vi "Global Stop Actions.vi"(7 "Command":T2=enum."Read", 8 "error in (no error)":errorcluster, 9 "Stop on Error?":bool, 10 "Stop?":bool, 11 "Stop Ref":T1) -> (0 "error out":errorcluster {"code" min=0 max=0}, 2 "Latched Stop":bool, 3 "Stop Ref out":T1)   [LabVIEW 2013, in "J1939 Addon Engine.lvlib" / "Stop FG.lvlib"]
uses:
  Stop FG.lvlib
  Stop Global Ref.ctl
  Stop Global Commands.ctl
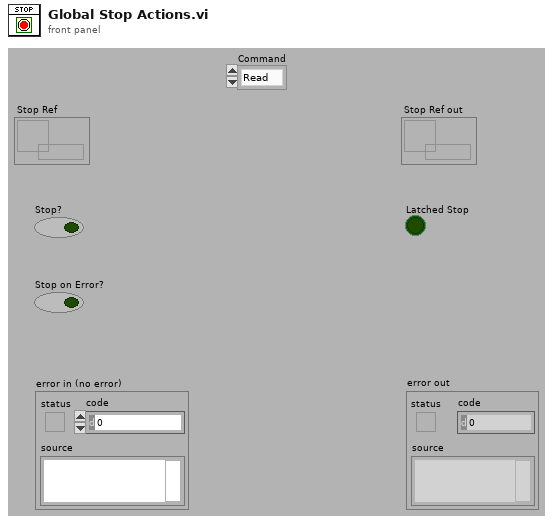
[diagram p1: front panel]
types:
  T1 = typedef "J1939 Addon Engine.lvlib/Stop FG.lvlib/Stop Global Ref.ctl" = refnum<data-value>
  T2 = typedef "J1939 Addon Engine.lvlib/Stop FG.lvlib/Stop Global Commands.ctl" = enum16{"Write", "Read", "Reset"}
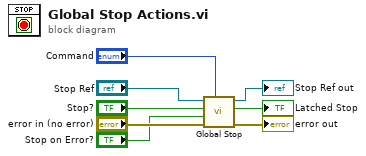
[diagram p0: block diagram]
diagram:
  n1 = call "Global Stop.vi"("Command"="Command", "error in (no error)"="error in (no error)", "Stop on Error?"="Stop on Error?", "Stop?"="Stop?", "Stop Ref"="Stop Ref") -> ("error out"=→"error out":errorcluster, "Latched Stop"=→"Latched Stop":bool, "Stop Ref out"=→"Stop Ref out":T1)  [unwired: 4 in]
